vi "Program03.vi"() -> ()   [LabVIEW 2020]
panel:
  out "Array":i32[](array[numeric])
  out "iteracje":i32
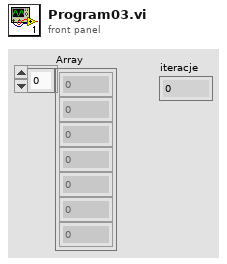
[diagram p1: front panel]
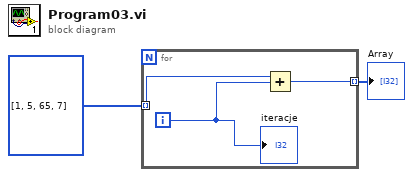
[diagram p0: block diagram]
diagram:
  n1 = for {
    tunnel: i32[] [1, 5, 65, 7] ("Array") -> [w4] mode=indexing
    tunnel: [w3] -> w1 mode=indexing
    i -> [w5]
    n2 = Add(x=w4, y=w5) -> (x+y=w3:i32)
    "iteracje" <- w5
  }
  "Array" <- w1
